vi "Get Security Count.vi"(8 "error in (no error)":errorcluster, 11 "VISA resource name":refnum<visa-resource-name>) -> (0 "error out":errorcluster, 2 "Security Count":i32, 3 "VISA resource name out":refnum<visa-resource-name>)   [LabVIEW 2017, in "Agilent 3352X Series.lvlib"]
doc: "Returns the security event count, which indicates if calibration or firmware have been changed or tampered.\n\nNote:\nThis VI is not supported by EDU33211A and EDU33212A."
uses:
  Doppia_Freq_Circuito/Agilent 3352X Series/Agilent 3352X Series.lvlib
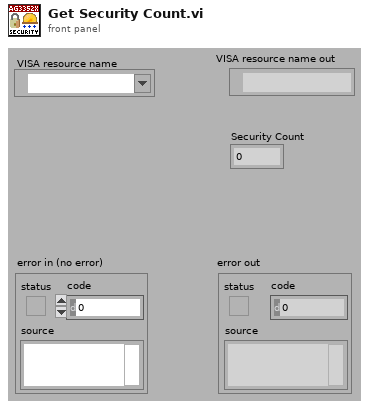
[diagram p1: front panel]
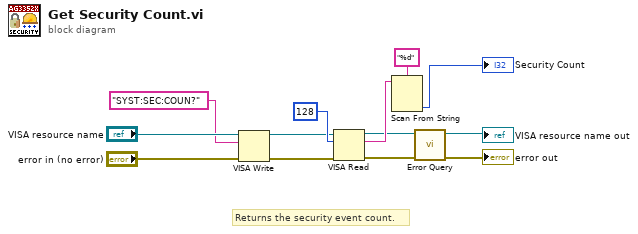
[diagram p0: block diagram]
diagram:
  # "Returns the security event count."
  n1 = VISA Write(VISA resource name="VISA resource name", write buffer="SYST:SEC:COUN?", error in (no error)="error in (no error)") -> (VISA resource name out=w10:refnum<visa-resource-name>, error out=w9:errorcluster)  [unwired: 1 out]
  n2 = VISA Read(VISA resource name=w10, byte count=u32 128, error in (no error)=w9) -> (VISA resource name out=w4:refnum<visa-resource-name>, read buffer=w7:string, error out=w3:errorcluster)  [unwired: 1 out]
  n3 = Scan From String(format string="%d", input string=w7) -> (output 1=→"Security Count":i32)  [unwired: 2 in, 4 out]
  n4 = call "Error Query.vi"("error in (no error)"=w3, "VISA resource name"=w4) -> ("error out"=→"error out":errorcluster, "VISA resource name out"=→"VISA resource name out":refnum<visa-resource-name>)  [unwired: 8 out]
